vi "setLegendAttribute.vi"(8 "Error In":errorcluster, 9 "on":bool, 10 "attribute":T1 items=["LegendNoAttribute"=0, "LegendShowLine"=1, "LegendShowSymbol"=2, "LegendShowBrush"=4], 11 "QwtPlotCurve In":refnum<class "QwtPlotCurve.lvclass">) -> (0 "Error Out":errorcluster, 3 "QwtPlotCurve Out":refnum<class "QwtPlotCurve.lvclass">)   [LabVIEW 2014, in "QwtPlotCurve.lvclass"]
doc: "LabVIEW-specific documentation is not yet available. See <b>https://qwt.sourceforge.io/class_qwt_plot_curve.html#setLegendAttribute</b>"
uses:
  QwtPlotCurve.lvclass
  LegendAttribute.ctl
  LQ Core/LQIdentity/LQIdentity.lvclass/LQIdentity.ctl
  LQ Core/LQ Core.lvlib
  LQ Core/LQIdentity/LQIdentity.lvclass
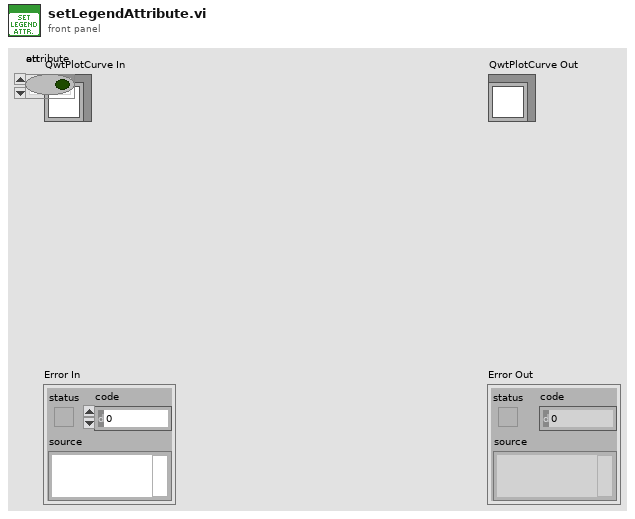
[diagram p1: front panel]
types:
  T1 = typedef "QwtPlotCurve.lvclass/LegendAttribute.ctl" = i32
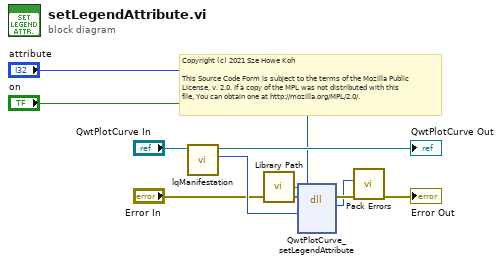
[diagram p0: block diagram]
diagram:
  # "Copyright (c) 2021 Sze Howe Koh\n\nThis Source Code Form is subject to the terms of the Mozilla Public\nLicense, v. 2.0. If a copy of the MPL was not distributed with this\nfile, You can obtain one at http://mozilla.org/MPL/2.0/."
  n1 = call "lqManifestation.vi"("LQIdentity in"="QwtPlotCurve In") -> ("Manifestation"=w7:u64, "LQIdentity out"=→"QwtPlotCurve Out":refnum<class "QwtPlotCurve.lvclass">)  [unwired: 9 in]
  n2 = call "Library Path.vi"() -> ("Library Path"=w8:path)
  n3 = dll-call lib="?" fn="QwtPlotCurve_setLegendAttribute"(path in=w8, error in="Error In", "_instance"=w7, "attribute"="attribute", "on"="on") -> (error out=w5:errorcluster, w3:i32)  [unwired: 4 in, 1 out]
  n4 = call "Pack Errors.vi"("Error In"=w5, "Error Code"=w3) -> ("Error Out"=→"Error Out":errorcluster)  [unwired: 9 in]
